vi "LVClass_Image get HASO sensor information.vi"(0 "Image in":refnum<class "Image.lvclass">, 11 "error in (no error)":errorcluster) -> (4 "Image out":refnum<class "Image.lvclass">, 6 "is_haso_image":bool, 8 "haso_serial_number":string, 15 "error out":errorcluster)   [LabVIEW 2020, in "Image.lvclass"]
doc: "Get metadata from Image object.\n\n--------------------------------------------------------------------------------\n\n<B>ImageIn </B> : Image object.\n<B>ImageOut </B> : Image object.\n<B>haso_serial_number </B> : Haso serial number.\n<B>camera_serial_number </B> : Camera serial number.\n<B>exposure_time_applied </B> : Exposure duration applied (us).\n<B>exposure_time_requested </B> : Exposure duration requested (us).\n<B>gain </B> : Applied gain (SI).\n<B>nb_summed_images </B> : Number of summed images.\n<B>is_smearing_removed </B> : Smearing_removed.\n<B>is_background_removed </B> : Background_removed.\n<B>trigger_type </B> : Trigger mode.\n<B>time_stamp </B> : Date of the acquired Image.\n<B>max_level </B> : Max level value.\n<B>comments </B> : Comments.\n<B>ErrorIn </B> : Error\n<B>ErrorOut </B> : Error\n\n--------------------------------------------------------------------------------"
uses:
  Image.lvclass
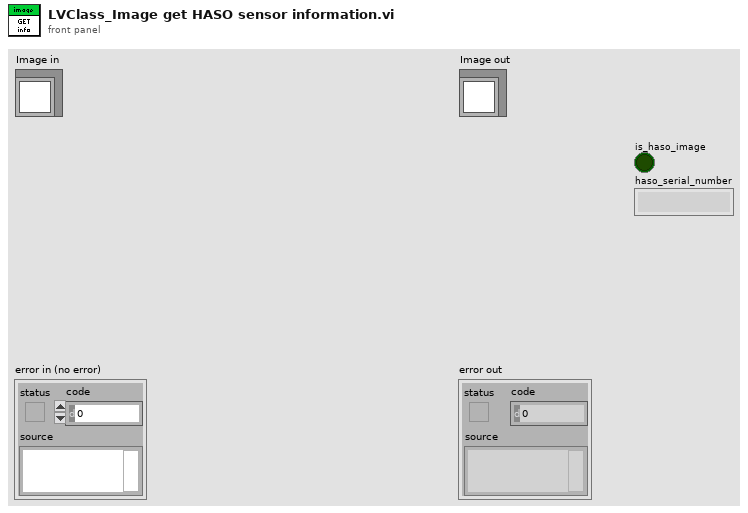
[diagram p1: front panel]
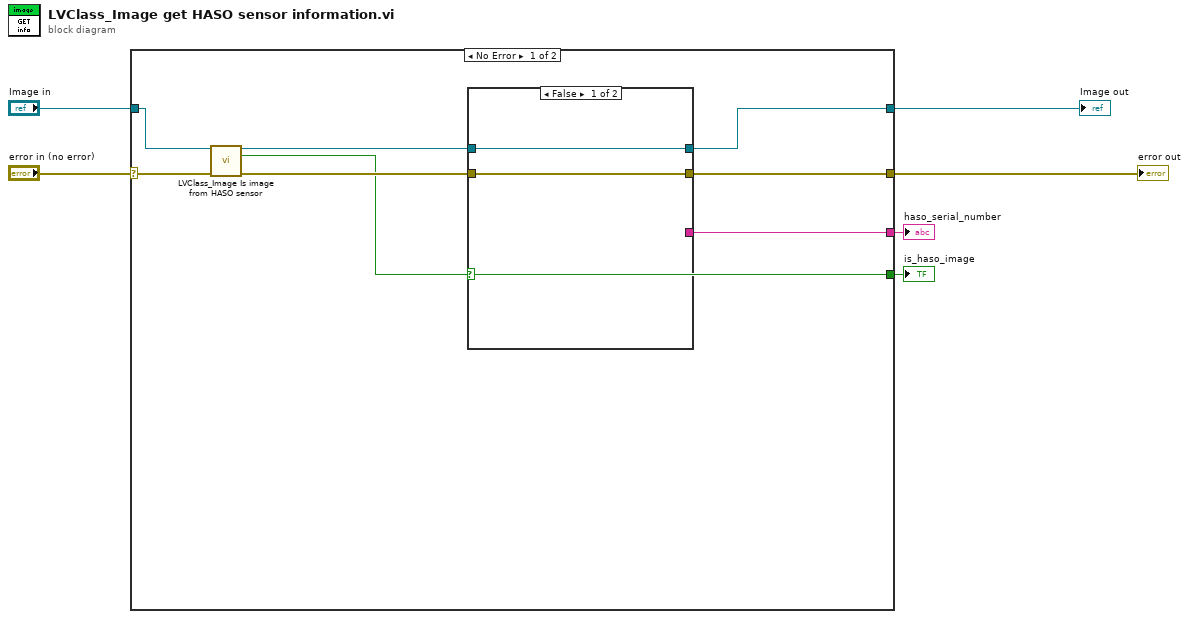
[diagram p0: block diagram]
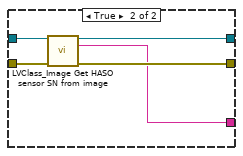
[diagram p2: hidden frame]
diagram:
  n1 = case shown="No Error" "error in (no error)" {
    selector: "error in (no error)" -> [w13 w23]
    tunnel: [w10 w23] -> w5
    tunnel: [w9 w22] -> w3
    tunnel: "Image in" -> [w14 w22]
    tunnel: [w7 _] -> w2
    tunnel: [w8 _] -> w1
    frame No Error {
      n2 = call "LVClass_Image Is image from HASO sensor.vi"("Image in"=w14, "error in (no error)"=w13) -> ("Image out"=w11:refnum<class "Image.lvclass">, "is_haso_image"=w7:bool, "error out"=w12:errorcluster)  [unwired: 11 in]
      n3 = case shown="False" w7 {
        tunnel: w12 -> [w15 w21]
        tunnel: w11 -> [w16 w20]
        tunnel: [w15 w19] -> w10
        tunnel: [w16 w18] -> w9
        tunnel: [_ w17] -> w8
        frame False {
        }
        frame True {
          n4 = call "LVClass_Image Get HASO sensor SN from image.vi"("Image in"=w20, "error in (no error)"=w21) -> ("Image out"=w18:refnum<class "Image.lvclass">, "haso_serial_number"=w17:string, "error out"=w19:errorcluster)  [unwired: 11 in]
        }
      }
    }
    frame Error {
    }
  }
  "error out" <- w5
  "Image out" <- w3
  "is_haso_image" <- w2
  "haso_serial_number" <- w1
